vi "_wmg_SelectItems2.vi"(10 "Item Syms":i32[](array[numeric]), 11 "Item name":string[](array[string])) -> (1 "Selected tem index":i32[](array[numeric]), 2 "Item Seleced?":bool, 3 "Selected tem":string[](array[string]))   [LabVIEW 2011]
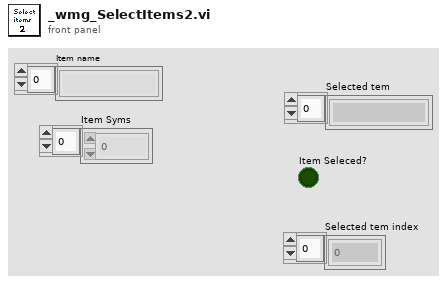
[diagram p1: front panel]
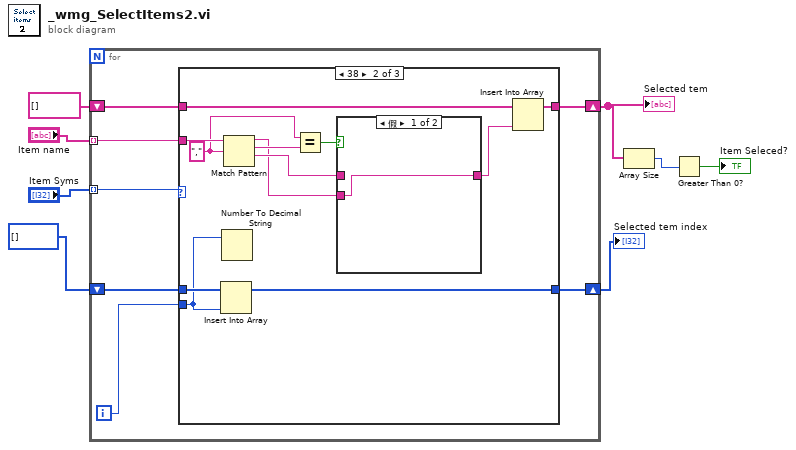
[diagram p0: block diagram]
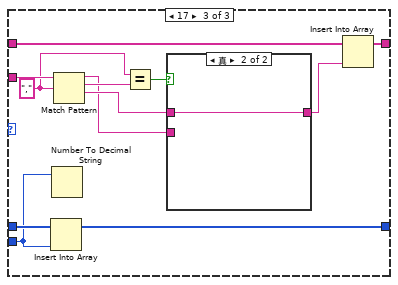
[diagram p4: hidden frame]
diagram:
  n1 = for {
    tunnel: "Item name" -> [w14] mode=indexing
    tunnel: "Item Syms" -> [w9] mode=indexing
    shift-right: [w13] -> w5
    shift-left: string[] [] ("Item name") -> [w15]
    shift-right: [w10] -> w1
    shift-left: i32[] [] ("Item Syms") -> [w12]
    i -> [w11]
    n2 = case shown="38" w9 {
      tunnel: w15 -> [w17 w29 w43]
      tunnel: w14 -> [_ w24 w38]
      tunnel: [w17 w26 w40] -> w13
      tunnel: w12 -> [w16 w28 w42]
      tunnel: w11 -> [_ w25 w39]
      tunnel: [w16 w27 w41] -> w10
      frame 37, Default {
      }
      frame 38 {
        w19 = "," ("正则表达式")
        n3 = Insert Into Array(array=w28, new element=w25) -> (w27:i32[])  [unwired: 1 in]
        n4 = Number To Decimal String(number=w25) -> ()  [unwired: 1 in, 1 out]
        n5 = Match Pattern(string=w24, regular expression=w19) -> (before substring=w18:string, match substring=w23:string, after substring=w21:string)  [unwired: 1 in, 1 out]
        n6 = Equal?(x=w19, y=w23) -> (x = y?=w22:bool)
        n7 = case shown="假" w22 {
          tunnel: w21 -> [_ w31]
          tunnel: [w30 w31] -> w20
          tunnel: w18 -> [w30 _]
          frame False {
          }
          frame True {
          }
        }
        n8 = Insert Into Array(array=w29, new element=w20) -> (w26:string[])  [unwired: 1 in]
      }
      frame 17 {
        w33 = "," ("正则表达式")
        n9 = Insert Into Array(array=w42, new element=w39) -> (w41:i32[])  [unwired: 1 in]
        n10 = Number To Decimal String(number=w39) -> ()  [unwired: 1 in, 1 out]
        n11 = Match Pattern(string=w38, regular expression=w33) -> (before substring=w32:string, match substring=w37:string, after substring=w35:string)  [unwired: 1 in, 1 out]
        n12 = Equal?(x=w33, y=w37) -> (x = y?=w36:bool)
        n13 = case shown="真" w36 {
          tunnel: w35 -> [_ w45]
          tunnel: [w44 w45] -> w34
          tunnel: w32 -> [w44 _]
          frame False {
          }
          frame True {
          }
        }
        n14 = Insert Into Array(array=w43, new element=w34) -> (w40:string[])  [unwired: 1 in]
      }
    }
  }
  "Selected tem" <- w5
  "Selected tem index" <- w1
  n15 = Array Size(array=w5) -> (size(s)=w3:i32)
  n16 = Greater Than 0?(x=w3) -> (x > 0?=→"Item Seleced?":bool)
